vi "write_key.vi"(8 "file_name":string, 10 "time":i64, 11 "key":string) -> ()   [LabVIEW 2017, in "Lib_code.lvlib"]
uses:
  Lib_code.lvlib
panel:
  out "输出簇":cluster{"key":string, "time":i64}
  in  "簇":cluster{"key":string, "time":i64}
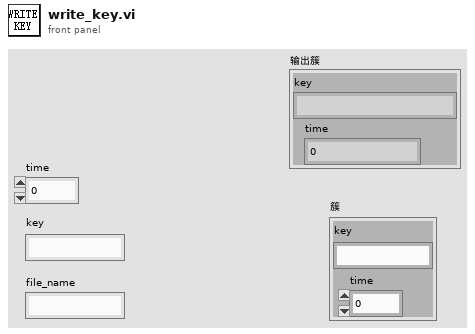
[diagram p1: front panel]
types:
  T1 = enum16{"big-endian, network order", "native, host order", "little-endian"}
  T2 = enum16{"open", "replace", "create", "open or create", "replace or create", "replace or create with confirmation"}
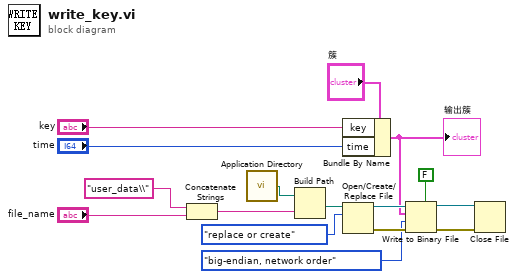
[diagram p0: block diagram]
diagram:
  n1 = Concatenate Strings("user_data\\" ("字符串"), "file_name") -> (w2:string)
  n2 = call <vilib>:"Application Directory.vi"() -> ("Application Directory"=w16:path)
  n3 = Build Path(base path=w16, name or relative path=w2) -> (appended path=w15:path)
  n4 = Bundle By Name(cluster="簇", "key"="key", "time"="time") -> (w8:cluster{"key":string, "time":i64})
  "输出簇" <- w8
  n5 = Open/Create/Replace File(file path (use dialog)=w15, operation (0:open)=T2."replace or create" ("操作(0:open)")) -> (refnum out=w13:refnum<file>, error out=w12:errorcluster)  [unwired: 4 in, 1 out]
  n6 = Write to Binary File(file (use dialog)=w13, data=w8, error in=w12, 5:FALSE ("预置数组或字符串大小？ (T)"), 9:T1."big-endian, network order" ("字节顺序(0:big-endian, network order)")) -> (refnum out=w11:refnum<file>, error out=w10:errorcluster)  [unwired: 1 in, 1 out]
  n7 = Close File(refnum=w11, error in=w10) -> ()  [unwired: 2 out]
